vi "Voltage Continuous Output.vi"() -> ()   [LabVIEW 2016]
doc: "This example demonstrates how to continuously generate an analog output waveform by providing new data to the output buffer as the task is running.\n\nThis example is useful if you want to generate a non-repeating waveform, make updates on-the-fly, or generate a frequency that is not an even divide-down of your sample clock. In this example, the default frequency value is 17 to demonstrate that non-regenerative output can be used to create a signal with a frequency that is not an even divide-down of your sample clock."
uses:
  <vilib>/Utility/error.llb/DialogType.ctl
  <vilib>/DAQmx/write.llb/DAQmx Write (Analog 1D Wfm NChan NSamp).vi
  <vilib>/DAQmx/create/channels.llb/DAQmx Create Channel (AO-Voltage-Basic).vi
  <vilib>/DAQmx/configure/timing.llb/DAQmx Timing (Sample Clock).vi
  <vilib>/DAQmx/miscellaneous.llb/DAQmx Fill In Error Info.vi
  <resource>/objmgr/daqmx.rc
  <vilib>/measure/NI_MABase.lvlib
panel:
  in  "Output Array":T1(array[cluster])=[{"Waveform Type"=4, "Amplitude"=1.5, "Frequency"=0.0}, {"Waveform Type"=0, "Amplitude"=1.0, "Frequency"=5.0}, {"Waveform Type"=0, "Amplitude"=2.0, "Frequency"=5.0}, {"Waveform Type"=0, "Amplitude"=3.0, "Frequency"=5.0}, {"Waveform Type"=0, "Amplitude"=4.0, "Frequency"=5.0}, {"Waveform Type"=0, "Amplitude"=5.0, "Frequency"=5.0}] {"Frequency" format="%0.2p"; "Amplitude" format="%0.2p"; "Waveform Type" items=["Sine Wave", "Triangle Wave", "Square Wave", "Sawtooth Wave", "Static"]}
  in  "Number of Samples":i32=5000
  in  "Stop":bool
  out "Waveform Graph":waveform(dbl)[](graph)=[{"t0"=timestamp(0 s since 1904-01-01), "dt"=4e-05, "Y"=array[5000 elements]}, {"t0"=timestamp(0 s since 1904-01-01), "dt"=4e-05, "Y"=array[5000 elements]}, {"t0"=timestamp(0 s since 1904-01-01), "dt"=4e-05, "Y"=array[5000 elements]}, {"t0"=timestamp(0 s since 1904-01-01), "dt"=4e-05, "Y"=array[5000 elements]}, {"t0"=timestamp(0 s since 1904-01-01), "dt"=4e-05, "Y"=array[5000 elements]}, {"t0"=timestamp(0 s since 1904-01-01), "dt"=4e-05, "Y"=array[5000 elements]}]
  in  "Sample Rate":dbl=25000.0
  in  "Sample Clock Source":tag="OnboardClock"
  in  "Max Voltage":dbl=5.0
  in  "Min Voltage":dbl=-5.0
  in  "Physical Channel(s)":tag="9264/ao0:5"
  out "Actual Sample Rate":dbl=25000.0 format="%0.2f"
  # "Channel Settings"
  # "Output"
  # "Timing and Buffer Settings"
  # "Waveform Settings"
  # "The number of elements in the waveform array\nmust equal the number of channels in the task."
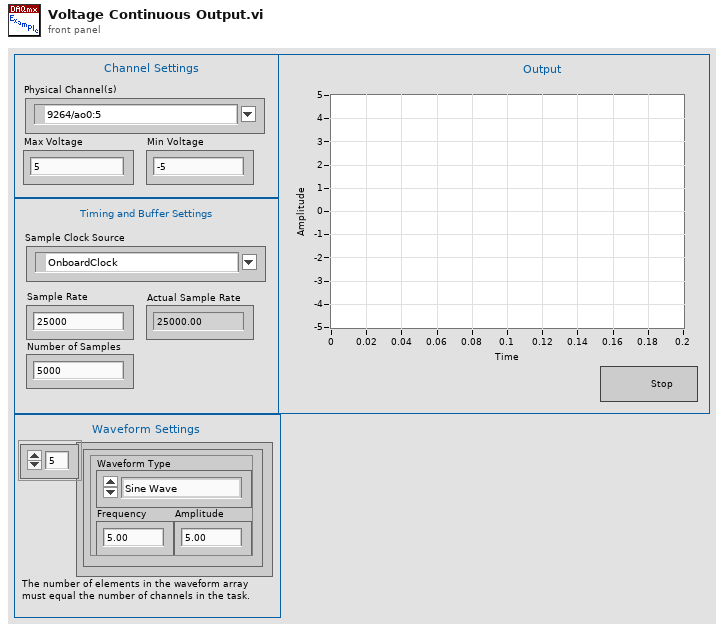
[diagram p1: front panel]
types:
  T1 = cluster{"Waveform Type":u16, "Amplitude":dbl, "Frequency":dbl}[]
  T2 = typedef "DialogType.ctl" = u16
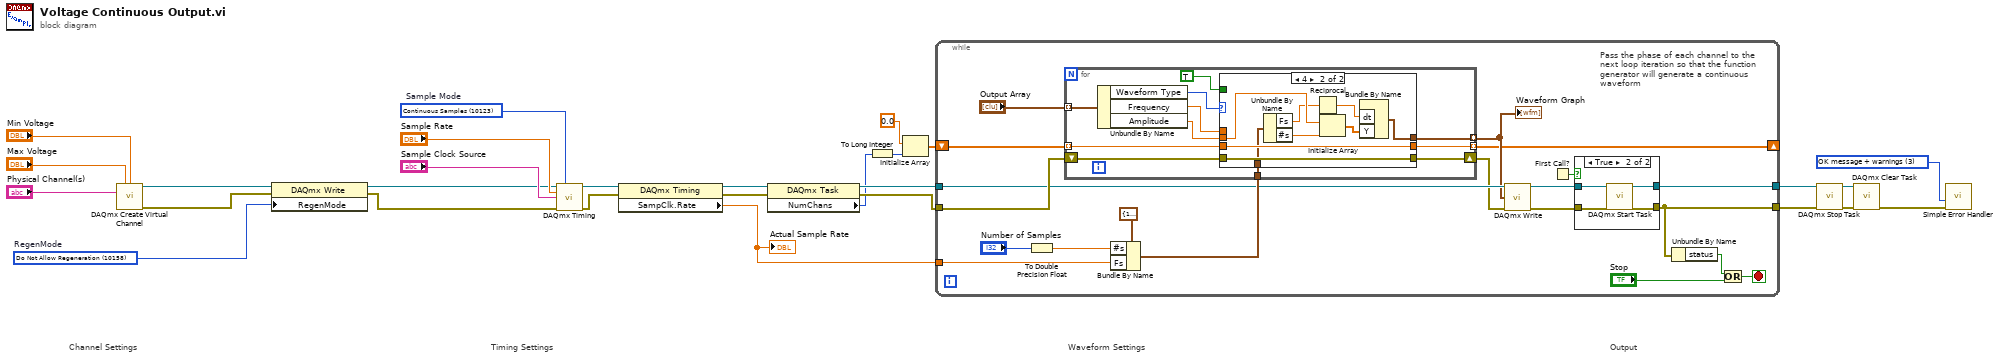
[diagram p0: block diagram]
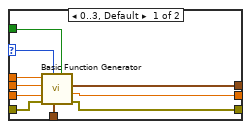
[diagram p3: hidden frame]
diagram:
  w11 = T2 3 items=["no dialog", "OK message", "continue or stop message", "OK message + warnings", "continue/stop + warnings"] ("type of dialog (OK msg:1)")
  w18 = 10158 items=["Allow Regeneration"=10097, "Do Not Allow Regeneration"=10158]  # RegenMode
  w28 = 10123 items=["Finite Samples"=10178, "Continuous Samples"=10123, "Hardware Timed Single Point"=12522]  # Sample Mode
  # "Output"
  # "Waveform Settings"
  # "Timing Settings"
  # "Channel Settings"
  n1 = call-poly <vilib>:"DAQmx Create Virtual Channel.vi"("maximum value"="Max Voltage", "minimum value"="Min Voltage", "physical channels"="Physical Channel(s)") -> ("task out"=w20:refnum<k21>, "error out"=w19:errorcluster)  [unwired: 11 in]
  n2 = property class="DAQmx Write"(reference=w20, error in=w19, "RegenMode"=w18) -> (reference out=w16:refnum<k21>, error out=w17:errorcluster)
  n3 = call-poly <vilib>:"DAQmx Timing.vi"("task/channels in"=w16, "sample mode"=w28, "rate"="Sample Rate", "source"="Sample Clock Source", "error in"=w17) -> ("task out"=w1:refnum<k21>, "error out"=w2:errorcluster)  [unwired: 9 in]
  n4 = property class="DAQmx Timing"(reference=w1, error in=w2) -> (reference out=w6:refnum<k21>, error out=w5:errorcluster, "SampClk.Rate"=w21:dbl)
  "Actual Sample Rate" <- w21
  n5 = property class="DAQmx Task"(reference=w6, error in=w5) -> (reference out=w8:refnum<k21>, error out=w7:errorcluster, "NumChans"=w4:u32)
  n6 = To Long Integer(number=w4) -> (32bit integer=w3:i32)
  n7 = Initialize Array(0.0 ("element"), w3) -> (w9:dbl[])
  n8 = while {
    tunnel: w7 -> [w48]
    tunnel: w21 -> [w46]
    tunnel: w8 -> [w44]
    tunnel: [w35] -> w13
    tunnel: [w34] -> w12
    shift-right: [w30] -> _
    shift-left: w9 -> [w29]
    stop <- w32 stop-if-true
    # "Pass the phase of each channel to the next loop iteration so that the function generator will generate a continuous waveform"
    n9 = To Double Precision Float(number="Number of Samples") -> (double precision float=w38:dbl)
    n10 = Bundle By Name(cluster=cluster{"Fs":dbl, "#s":dbl} {"Fs"=1000.0, "#s"=1000.0} ("sampling info"), "#s"=w38, "Fs"=w46) -> (w45:cluster{"Fs":dbl, "#s":dbl})
    n11 = for {
      tunnel: w45 -> [w64]
      tunnel: "Output Array" -> [w62] mode=indexing
      tunnel: [w59] -> w39 mode=indexing
      tunnel: [w58] -> w30 mode=indexing
      tunnel: w29 -> [w56] mode=indexing
      shift-right: [w63] -> w41
      shift-left: w48 -> [w65]
      n12 = Unbundle By Name(w62) -> ("Waveform Type"=w55:u16, "Frequency"=w61:dbl, "Amplitude"=w60:dbl)
      n13 = case shown="4" w55 {
        selector: w55 -> [w66 _]
        tunnel: w65 -> [w75 w83]
        tunnel: w64 -> [w74 w81]
        tunnel: [w73 w83] -> w63
        tunnel: w61 -> [w72 _]
        tunnel: w60 -> [w71 w82]
        tunnel: [w70 w79] -> w59
        tunnel: [w69 w84] -> w58
        tunnel: TRUE ("reset signal") -> [w68 _]
        tunnel: w56 -> [w67 w84]
        frame 0..3, Default {
          n14 = call <vilib>:"Basic Function Generator.vi"("reset signal"=w68, "sampling info"=w74, "signal type"=w66, "error in (no error)"=w75, "phase"=w67, "amplitude"=w71, "frequency"=w72) -> ("error out"=w73:errorcluster, "phase out"=w69:dbl, "signal out"=w70:waveform(dbl))  [unwired: 2 in]
        }
        frame 4 {
          n15 = Unbundle By Name(w81) -> ("Fs"=w76:dbl, "#s"=w78:dbl)
          n16 = Reciprocal(x=w76) -> (1/x=w77:dbl)
          n17 = Initialize Array(w82, w78) -> (w80:dbl[])
          n18 = Bundle By Name("dt"=w77, "Y"=w80) -> (w79:waveform(dbl))  [unwired: 1 in]
        }
      }
    }
    "Waveform Graph" <- w39
    n19 = call-poly <vilib>:"DAQmx Write.vi"("task/channels in"=w44, "data"=w39, "error in"=w41) -> ("task out"=w43:refnum<k21>, "error out"=w42:errorcluster)  [unwired: 10 in, 1 out]
    n20 = First Call?() -> (First Call?: T/F=w36:bool)
    n21 = case shown="True" w36 {
      tunnel: w43 -> [w49 w54]
      tunnel: w42 -> [w50 w53]
      tunnel: [w49 w52] -> w35
      tunnel: [w50 w51] -> w34
      frame False {
      }
      frame True {
        n22 = call <vilib>:"DAQmx Start Task.vi"("task/channels in"=w54, "error in"=w53) -> ("task out"=w52:refnum<k21>, "error out"=w51:errorcluster)  [unwired: 12 in]
      }
    }
    n23 = Unbundle By Name(w34) -> ("status"=w31:bool)
    n24 = Or(x=w31, y="Stop") -> (x .or. y?=w32:bool)
  }
  n25 = call <vilib>:"DAQmx Stop Task.vi"("task/channels in"=w13, "error in"=w12) -> ("task out"=w15:refnum<k21>, "error out"=w14:errorcluster)  [unwired: 12 in]
  n26 = call <vilib>:"DAQmx Clear Task.vi"("task in"=w15, "error in"=w14) -> ("error out"=w27:errorcluster)  [unwired: 13 in]
  n27 = call <vilib>:"Simple Error Handler.vi"("type of dialog (OK msg:1)"=w11, "error in (no error)"=w27) -> ()  [unwired: 3 in, 5 out]
